vi "Tutorial coke machine.vi"() -> ()   [LabVIEW 2015]
panel:
  out "Money Deposited":string
  out "Dispense Coke":bool
  in  "Nickel":bool
  in  "Dime":bool
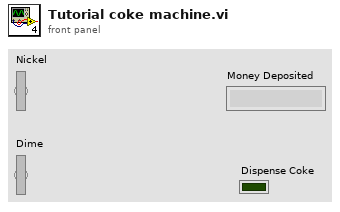
[diagram p1: front panel]
types:
  T1 = enum16{"Start", "5 cents", "10 cents", "Dispense"}
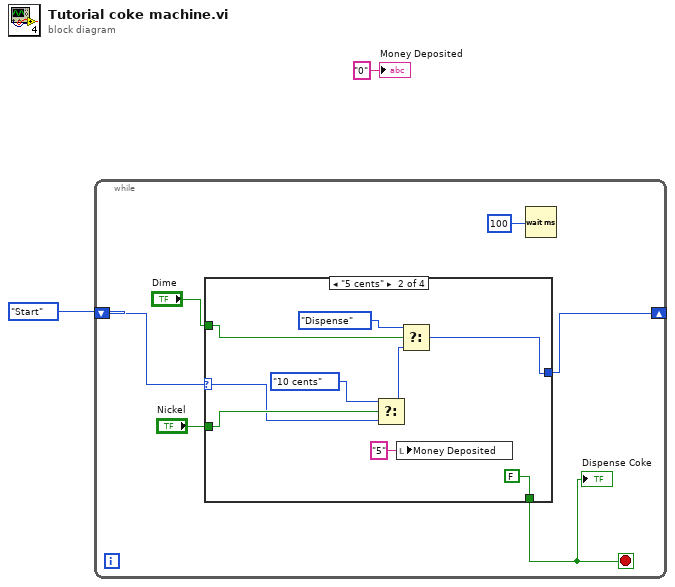
[diagram p0: block diagram]
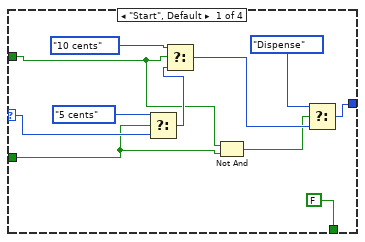
[diagram p2: hidden frame]
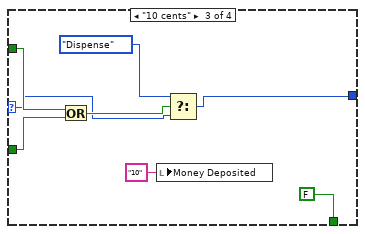
[diagram p3: hidden frame]
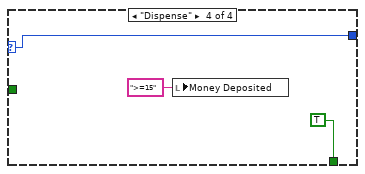
[diagram p4: hidden frame]
diagram:
  n1 = while {
    shift-right: [w5] -> _
    shift-left: T1."Start" -> [w8]
    stop <- w4 stop-if-true
    n2 = case shown="\"5 cents\"" w8 {
      selector: w8 -> [w17 w23 w31 w38]
      tunnel: "Dime" -> [w13 w27 w36 _]
      tunnel: "Nickel" -> [w12 w24 w35 _]
      tunnel: [w10 w21 w30 w38] -> w5
      tunnel: [FALSE FALSE FALSE TRUE] -> w4
      frame "Start", Default {
        n3 = Select(t=T1."5 cents", s=w12, f=w17) -> (s? t:f=w16:T1)
        n4 = Select(t=T1."10 cents", s=w13, f=w16) -> (s? t:f=w15:T1)
        n5 = Not And(1:w12, 2:w13) -> (0:w11:bool)
        n6 = Select(t=T1."Dispense", s=w11, f=w15) -> (s? t:f=w10:T1)
      }
      frame "5 cents" {
        n7 = Select(t=T1."10 cents", s=w24, f=w23) -> (s? t:f=w22:T1)
        n8 = local write "Money Deposited"("5" ("Money Deposited")) -> ()
        n9 = Select(t=T1."Dispense", s=w27, f=w22) -> (s? t:f=w21:T1)
      }
      frame "10 cents" {
        n10 = Or(x=w36, y=w35) -> (x .or. y?=w33:bool)
        n11 = local write "Money Deposited"("10" ("Money Deposited")) -> ()
        n12 = Select(t=T1."Dispense", s=w33, f=w31) -> (s? t:f=w30:T1)
      }
      frame "Dispense" {
        n13 = local write "Money Deposited"(">=15" ("Money Deposited")) -> ()
      }
    }
    "Dispense Coke" <- w4
    n14 = Wait (ms)(milliseconds to wait=u32 100 ("millisecond timer value")) -> ()  [unwired: 1 out]
  }
  "Money Deposited" <- "0" ("Money Deposited")
